vi "CreateLog.vi"(8 "error in (no error)":errorcluster, 11 "EventLoggerData in":T1) -> (0 "error out":errorcluster, 3 "EventLoggerData out":T1)   [LabVIEW 2019, in "EventLogger.lvlib"]
uses:
  EventLogger.lvlib
  Cluster - EventLoggerData.ctl
  <vilib>/Utility/sysdir.llb/System Directory Type.ctl
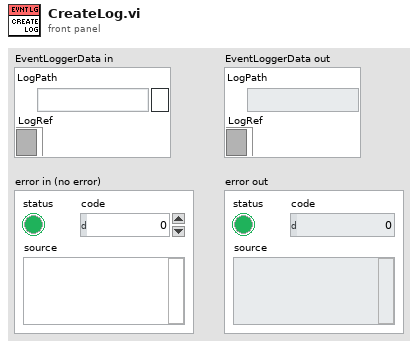
[diagram p1: front panel]
types:
  T1 = typedef "EventLogger.lvlib/Cluster - EventLoggerData.ctl" = cluster{"LogPath":path, "LogRef":refnum<file>}
  T2 = enum16{"open", "replace", "create", "open or create", "replace or create", "replace or create with confirmation"}
  T3 = typedef "System Directory Type.ctl" = i32
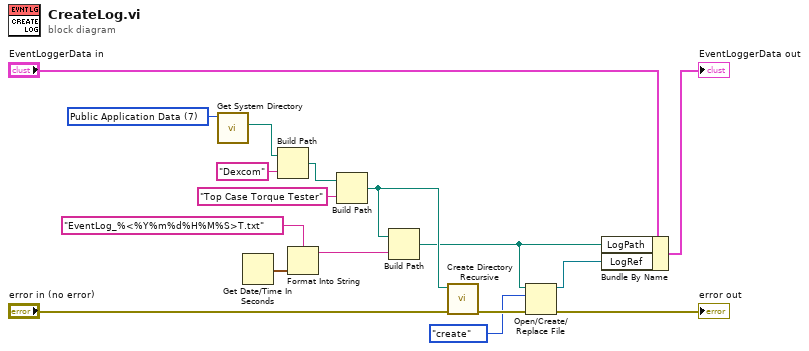
[diagram p0: block diagram]
diagram:
  w15 = T3 7 items=["User Home"=0, "User Desktop"=1, "User Documents"=2, "User Application Data"=3, "User Preferences"=4, "User Temporary"=5, "Public Documents"=6, "Public Application Data"=7, "Public Preferences"=8, "Public Cache"=13, "System Core Libraries"=9, "System Installed Libraries"=10, "Application Files"=11, "Boot Volume Root"=12] ("system directory type")
  n1 = call <vilib>:"Get System Directory.vi"("system directory type"=w15) -> ("system directory"=w14:path)  [unwired: 10 in]
  n2 = Get Date/Time In Seconds() -> (seconds since 1Jan1904=w9:timestamp)
  n3 = Build Path(base path=w14, name or relative path="Dexcom") -> (appended path=w12:path)
  n4 = Format Into String(format string="EventLog_%<%Y%m%d%H%M%S>T.txt", w9) -> (resulting string=w8:string)  [unwired: 2 in, 1 out]
  n5 = Build Path(base path=w12, name or relative path="Top Case Torque Tester") -> (appended path=w6:path)
  n6 = Build Path(base path=w6, name or relative path=w8) -> (appended path=w1:path)
  n7 = call <vilib>:"Create Directory Recursive.vi"("error in (no error)"="error in (no error)", "directory"=w6) -> ("error out"=w7:errorcluster)  [unwired: 3 in, 2 out]
  n8 = Open/Create/Replace File(file path (use dialog)=w1, error in=w7, operation (0:open)=T2."create") -> (refnum out=w2:refnum<file>, error out=→"error out":errorcluster)  [unwired: 3 in, 1 out]
  n9 = Bundle By Name(cluster="EventLoggerData in", "LogPath"=w1, "LogRef"=w2) -> (→"EventLoggerData out":T1)
